vi "GOOP_MyComputer_Interface_CreateNewWizard_Invoke.vi"(10 "New Item Parent":T1, 11 "Wizard":u64) -> (3 "Canceled":bool)   [LabVIEW 2020]
uses:
  <resource>/Framework/Providers/API/mxLvNIIM.ctl
  SubVIs/GOOP_ClassProviderClassType.ctl
  ClassProviders/Provider_BaseClassInterface/ClassWriter_class/ClassWriter.lvclass
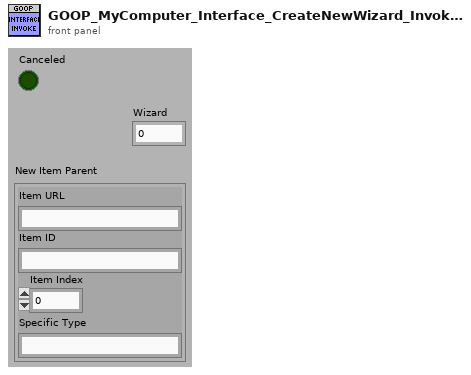
[diagram p1: front panel]
types:
  T1 = typedef "mxLvNIIM.ctl" = cluster{"Item URL":string, "Item ID":string, "Item Index":i32, "Specific Type":string}
  T2 = typedef "GOOP_ClassProviderClassType.ctl" = enum16{"ClassWriter", "ClassReader"}
  T3 = typedef "ClassWriter.lvclass/CreateInterfaceData.ctl" = cluster{"InterfaceName":string, "InterfaceFolder":path, "InterfaceDescription":string, "FolderSuffix":string, "MethodsToCreate":T4[], "ParentInterfaces":path[]}
  T4 = typedef "ClassWriter.lvclass/InterfaceMethodsToCreate.ctl" = cluster{"Name":string, "Description":string, "MethodsArgumentsIn":T5[], "MethodsArgumentsOut":T5[], "DecendantsMustOverride":bool}
  T5 = typedef "CommonVIs_AttributeType.ctl" = cluster{"Name":string, "DataType":T6, "ArrayDim":i32, "CtrlPath":path, "DataTypeString":string, "AccessScope":T7, "InitialData":variant}
  T6 = typedef "CommonVIs_AttributeDataType.ctl" = enum16{"UINT8", "INT8", "UINT16", "INT16", "UINT32", "INT32", "UINT64", "INT64", "SGL", "DBL", "EXT", "CSG", "CDB", "CXT", "TimeStamp", "STRING", "PATH", "BOOL", "ENUM", "RefNum", "VIRefNum", "LabVIEW Class", "Cluster", "Variant", "TypeDef", "Waveform", "LabVIEW Object", "Other", "void", "Set", "Map"}
  T7 = typedef "GDSString_AccessScopeModifierType.ctl" = enum16{"public", "private", "protected", "internal"}
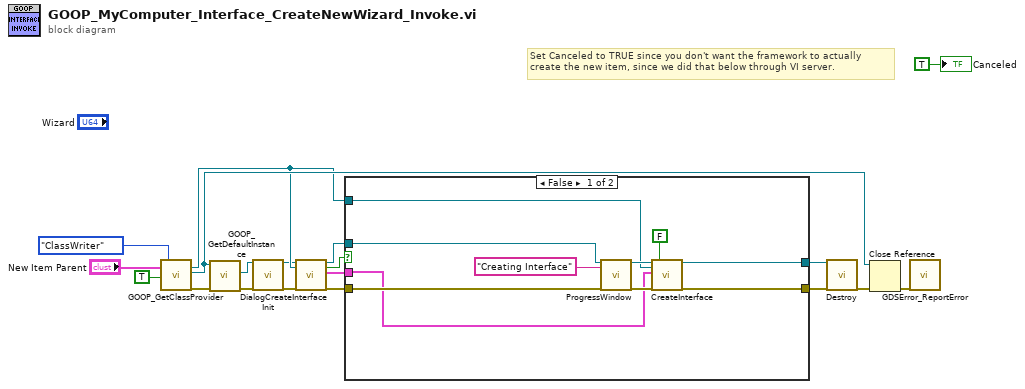
[diagram p0: block diagram]
diagram:
  # "Set Canceled to TRUE since you don't want the framework to actually\ncreate the new item, since we did that below through VI server."
  n1 = call "GOOP_GetClassProvider.vi"("New Item Parent/Object"="New Item Parent", "CreateClass"=TRUE, "ProviderClassType"=GOOP_ClassProviderClassType."ClassWriter") -> ("ProjectItem"=w13:refnum<vi>, "LVClass.Open"=w17:refnum<vi>, "error out"=w4:errorcluster)  [unwired: 14 in]
  n2 = call "GOOP_GetDefaultInstance.vi"("error in"=w4, "LVClassIn"=w17) -> ("error out"=w5:errorcluster, "ClassWriter.lvclass"=w3:refnum<class "ClassWriter.lvclass">)  [unwired: 7 in, 1 out]
  n3 = call-dynamic "Init.vi"("ClassWriter in"=w3, "error in (no error)"=w5) -> ("ClassWriter out"=w7:refnum<class "ClassWriter.lvclass">, "error out"=w6:errorcluster)  [unwired: 16 in]
  n4 = call-dynamic "DialogCreateInterface.vi"("ClassWriter in"=w7, "ProjectItem Refnum"=w13, "error in (no error)"=w6) -> ("ClassWriter out"=w15:refnum<class "ClassWriter.lvclass">, "Cancelled"=w14:bool, "CreateInterfaceData"=w2:T3, "error out"=w16:errorcluster)  [unwired: 13 in]
  n5 = case shown="False" w14 {
    tunnel: w15 -> [w29 w30]
    tunnel: w16 -> [w28 w31]
    tunnel: w13 -> [w25 _]
    tunnel: [w22 w31] -> w11
    tunnel: [w21 w30] -> w12
    tunnel: w2 -> [w23 _]
    frame False {
      n6 = call-dynamic "ProgressWindow.vi"("ClassWriter in"=w29, "Message(Exit)"="Creating Interface", "error in (no error)"=w28) -> ("ClassWriter out"=w27:refnum<class "ClassWriter.lvclass">, "error out"=w26:errorcluster)  [unwired: 15 in]
      n7 = call-dynamic "CreateInterface.vi"("ClassWriter.lvclass"=w27, "ProjectTreePosition(String or Project Item Ref)"=w25, "CreateInterfaceData"=w23, "error in (no error)"=w26, "KeepLvClassRefOpen(False)"=FALSE) -> ("ClassWriter.lvclass"=w21:refnum<class "ClassWriter.lvclass">, "error out"=w22:errorcluster)  [unwired: 12 in, 1 out]
    }
    frame True {
    }
  }
  n8 = call-dynamic "Destroy.vi"("ClassWriter.lvclass"=w12, "error in (no error)"=w11) -> ("error out"=w18:errorcluster)  [unwired: 17 in]
  n9 = Close Reference(reference=w17, error in (no error)=w18) -> (error out=w1:errorcluster)
  n10 = call "GDSError_ReportError.vi"("error in (no error)"=w1) -> ()  [unwired: 18 in, 1 out]
  "Canceled" <- TRUE ("Canceled")
